vi "250224_Nikon_Control.vi"() -> ()   [LabVIEW 2014]
doc: "This simple VI control few elements of a Nikon Ti2 microscope.\nAny kind of supplementary element can be controlled with a new event type (flurorescence cube turret for example)"
panel:
  in  "Cluster commandes":T1={"Dia lamp"=TRUE, "Dia lamp intensity"=1689.1304347826087, "Objective"=2, "Light path"=2, "Z pos (µm)"=335593, "Filter wheel 2"=2, "Filter wheel 1"=2, "Shutter 2"=TRUE, "Shutter 1"=TRUE} {"Filter wheel 1" items=["1"=1, "2"=2, "3"=3, "4"=4, "5"=5, "6"=6]; "Filter wheel 2" items=["1"=1, "2"=2, "3"=3, "4"=4, "5"=5, "6"=6]; "Z pos (µm)" min=0 max=990000 step=100 scale=0.0..990000.0; "Light path" items=["1- Eyepiece"=1, "2- Right"=2, "3- Left + Eyepiece"=3, "4- Left"=4]; "Objective" items=["1- PLAN APO 100X 1,45 Oil"=1, "2- Empty"=2, "3- Empty"=3, "4- Empty"=4, "5- Empty"=5, "6- Empty"=6]; "Dia lamp intensity" scale=0.0..2100.0}
  out "Cluster µscope":T2
  in  "stop":bool
  in  "NikonTi2AxLib.INikonTi2AxMicroscope":refnum<k7>
  out "error out":errorcluster={"status"=TRUE, "code"=-9, "source"="Exception occured in Nikon.Ti2.Microscope.1: Failed in 231026_NikonTi2_Indicators_v2.vi"} caption="sortie d'erreur"
  in  "error in":errorcluster caption="entrée d'erreur"
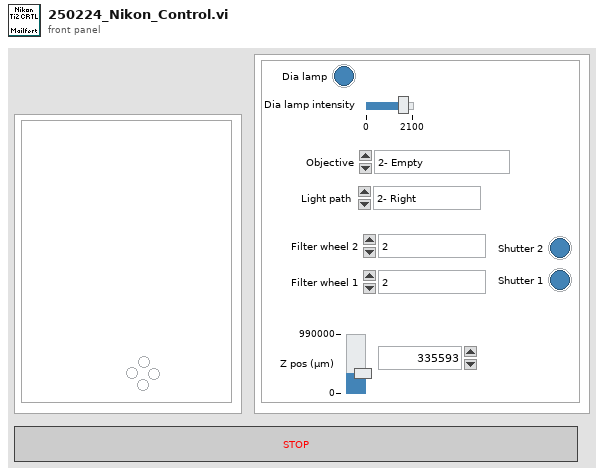
[diagram p1: front panel]
types:
  T1 = cluster{"Dia lamp":bool, "Dia lamp intensity":dbl, "Objective":i32, "Light path":u32, "Z pos (µm)":i32, "Filter wheel 2":u32, "Filter wheel 1":u32, "Shutter 2":bool, "Shutter 1":bool}
  T2 = cluster{"Eyepiece":bool, "Right":bool, "Left + Eyepiece":bool, "Left":bool}
  T3 = cluster{"iNOSEPIECE":i32, "iLIGHTPATH":i32, "iDIA_LAMP_Switch":i32, "iDIA_LAMP_Pos":i32, "iZPOSITION":i32, "iPFS_SWITCH":i32, "iPFS_STATUS":i32, "iPFS_OFFSET":i32, "iTURRET2POS":i32, "Turret2SHUTTER":i32, "iTURRET1POS":i32, "Turret1SHUTTER":i32}
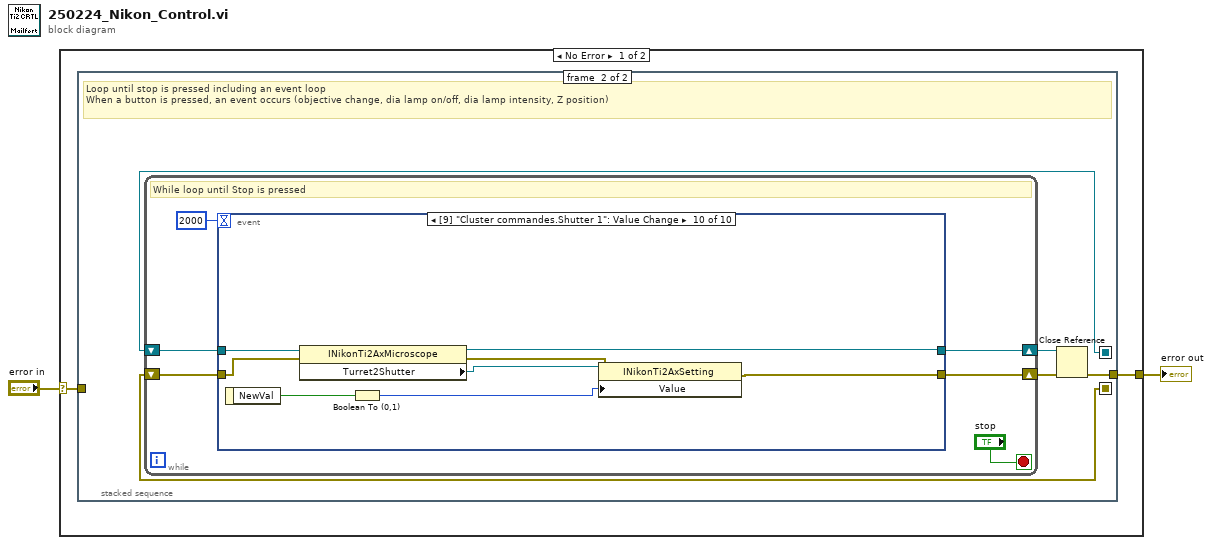
[diagram p0: block diagram]
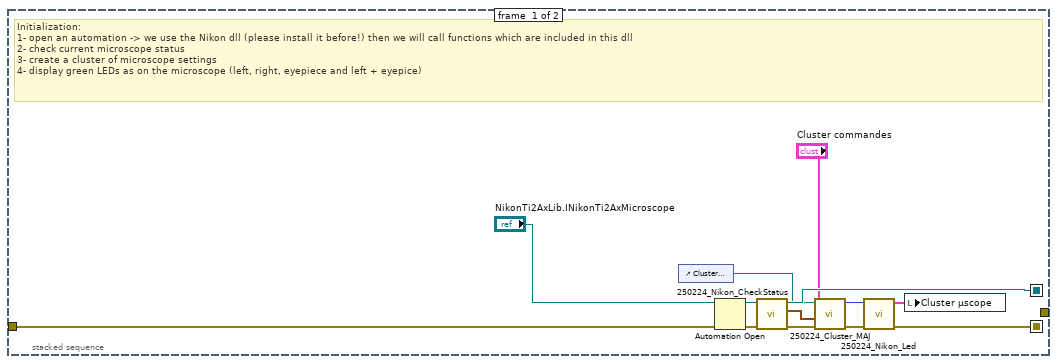
[diagram p2: hidden frame]
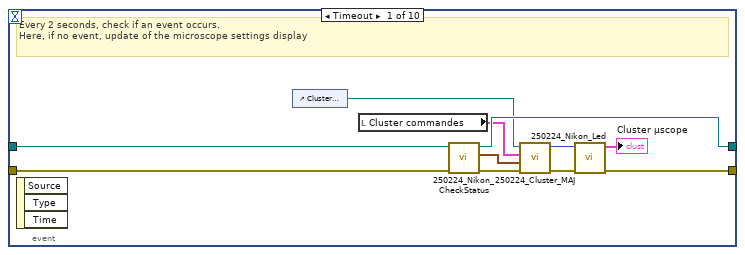
[diagram p3: hidden frame]
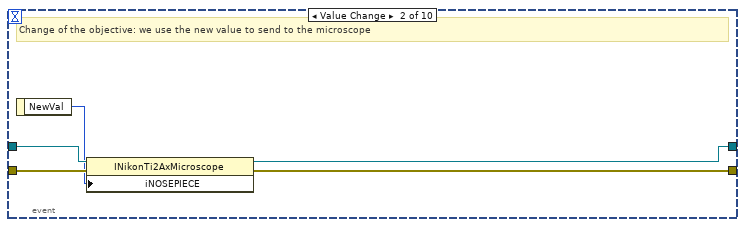
[diagram p4: hidden frame]
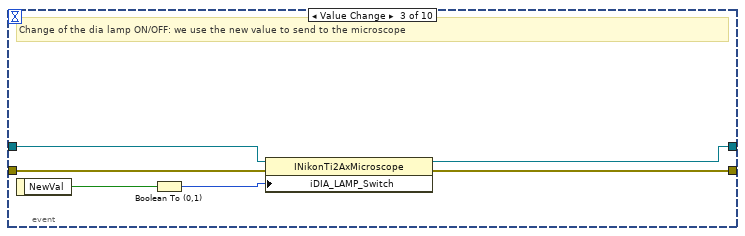
[diagram p5: hidden frame]
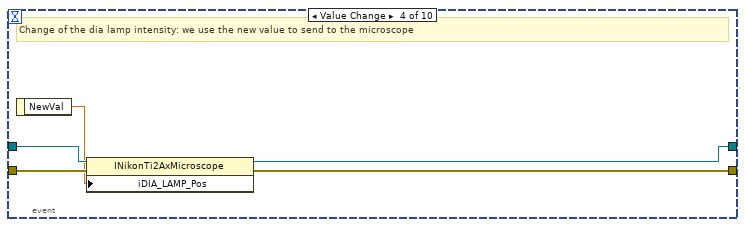
[diagram p6: hidden frame]
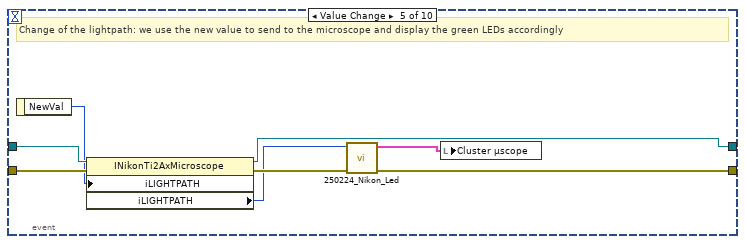
[diagram p7: hidden frame]
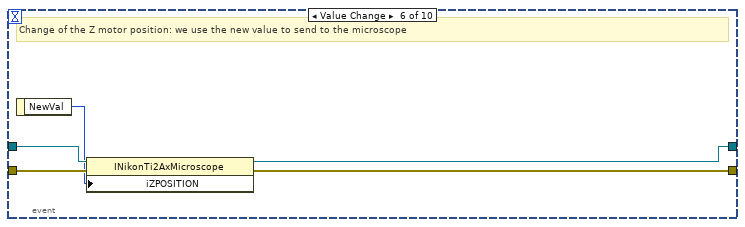
[diagram p8: hidden frame]
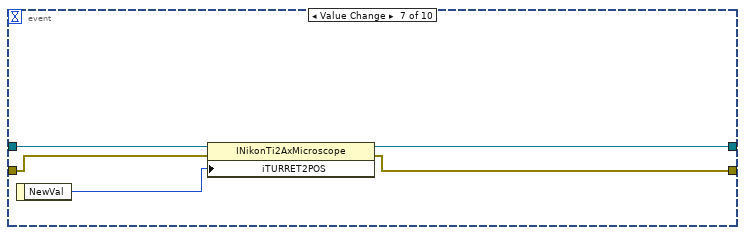
[diagram p9: hidden frame]
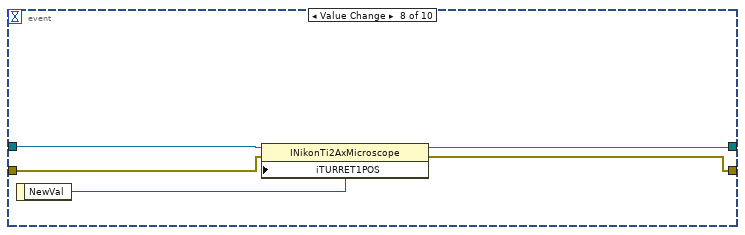
[diagram p10: hidden frame]
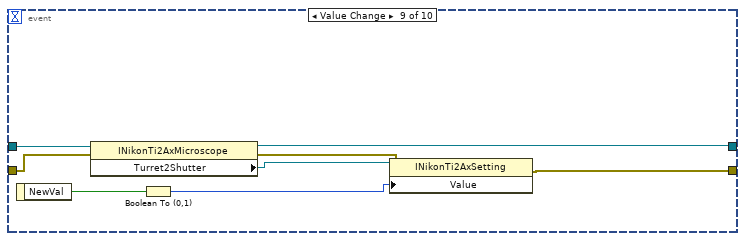
[diagram p11: hidden frame]
diagram:
  n1 = case shown="No Error" "error in" {
    selector: "error in" -> [w4 w95]
    tunnel: [w3 w95] -> w1
    frame No Error {
      n2 = stacked-sequence {
        seq-local: [w13 _] -> [_ w22]
        seq-local: [w7 _] -> [_ w18]
        tunnel: w4 -> [w14 _]
        tunnel: [_ w19] -> w3
        frame #0 {
          # "Initialization:\n1- open an automation -> we use the Nikon dll (please install it before!) then we will call functions which are included in this dll\n2- check current microscope status\n3- create a cluster of microscope settings\n4- display green LEDs as on the microscope (left, right, eyepiece and left + eyepice)"
          n3 = control-ref of="Cluster commandes"() -> (w6:refnum<vi>)
          n4 = Automation Open(error in (no error)=w14, Automation Refnum="NikonTi2AxLib.INikonTi2AxMicroscope") -> (Automation Refnum=w16:refnum<k7>, error out=w15:errorcluster)  [unwired: 2 in]
          n5 = call "250224_Nikon_CheckStatus.vi"("error in"=w15, "NikonTi2AxLib.INikonTi2AxMicroscope"=w16) -> ("error out"=w9:errorcluster, "Nikon status cluster"=w12:T3, "reference out"=w13:refnum<k7>)  [unwired: 7 in]
          n6 = call "250224_Cluster_MAJ.vi"("error in (no error)"=w9, "Nikon status cluster"=w12, 10:"Cluster commandes"="Cluster commandes", 11:"Cluster commandes"=w6) -> ("error out"=w8:errorcluster, "iLIGHTPATH"=w10:i32)  [unwired: 6 in]
          n7 = call "250224_Nikon_Led.vi"("error in"=w8, "Light path"=w10) -> ("error out"=w7:errorcluster, "Cluster µscope"=w11:T2)  [unwired: 8 in]
          n8 = local write "Cluster µscope"(w11) -> ()
        }
        frame #1 {
          # "Loop until stop is pressed including an event loop\nWhen a button is pressed, an event occurs (objective change, dia lamp on/off, dia lamp intensity, Z position)"
          n9 = while {
            shift-right: [w23] -> w20
            shift-left: w18 -> [w28]
            shift-right: [w24] -> w21
            shift-left: w22 -> [w25]
            stop <- "stop" stop-if-true
            # "While loop until Stop is pressed"
            n10 = event shown="[9] \"Cluster commandes.Shutter 1\": Value Change" {
              selector: _ -> [_ _ _ _ _ _ _ _ _ _]
              dyn-events: _ -> [_ _ _ _ _ _ _ _ _ _]
              timeout: 2000 -> [_ _ _ _ _ _ _ _ _ _]
              tunnel: [w36 w41 w47 w52 w60 w67 w70 w74 w81 w89] -> w23
              tunnel: w28 -> [w39 w43 w49 w54 w61 w65 w71 w77 w86 w94]
              tunnel: w25 -> [w38 w44 w50 w55 w62 w66 w73 w78 w85 w93]
              tunnel: [w37 w42 w48 w53 w63 w68 w69 w75 w82 w90] -> w24
              event Timeout {
                # "Every 2 seconds, check if an event occurs.\nHere, if no event, update of the microscope settings display"
                n11 = event-data() -> ()  [unwired: 1 in, 3 out]
                n12 = control-ref of="Cluster commandes"() -> (w29:refnum<vi>)
                n13 = local read "Cluster commandes"() -> (w30:T1)
                n14 = call "250224_Nikon_CheckStatus.vi"("error in"=w39, "NikonTi2AxLib.INikonTi2AxMicroscope"=w38) -> ("error out"=w33:errorcluster, "Nikon status cluster"=w34:T3, "reference out"=w37:refnum<k7>)  [unwired: 7 in]
                n15 = call "250224_Cluster_MAJ.vi"("error in (no error)"=w33, "Nikon status cluster"=w34, 10:"Cluster commandes"=w30, 11:"Cluster commandes"=w29) -> ("error out"=w32:errorcluster, "iLIGHTPATH"=w31:i32)  [unwired: 6 in]
                n16 = call "250224_Nikon_Led.vi"("error in"=w32, "Light path"=w31) -> ("error out"=w36:errorcluster, "Cluster µscope"=→"Cluster µscope":T2)  [unwired: 8 in]
              }
              event "Cluster commandes.Objective": Value Change {
                # "Change of the objective: we use the new value to send to the microscope"
                n17 = event-data() -> ("NewVal"=w40:i32)  [unwired: 1 in]
                n18 = property class="INikonTi2AxMicroscope"(reference=w44, error in=w43, "iNOSEPIECE"=w40) -> (reference out=w42:refnum<k7>, error out=w41:errorcluster)
              }
              event "Cluster commandes.Dia lamp": Value Change {
                # "Change of the dia lamp ON/OFF: we use the new value to send to the microscope"
                n19 = event-data() -> ("NewVal"=w46:bool)  [unwired: 1 in]
                n20 = Boolean To (0,1)(Boolean=w46) -> (0, 1=w45:i16)
                n21 = property class="INikonTi2AxMicroscope"(reference=w50, error in=w49, "iDIA_LAMP_Switch"=w45) -> (reference out=w48:refnum<k7>, error out=w47:errorcluster)
              }
              event "Cluster commandes.Dia lamp intensity": Value Change {
                # "Change of the dia lamp intensity: we use the new value to send to the microscope"
                n22 = event-data() -> ("NewVal"=w51:dbl)  [unwired: 1 in]
                n23 = property class="INikonTi2AxMicroscope"(reference=w55, error in=w54, "iDIA_LAMP_Pos"=w51) -> (reference out=w53:refnum<k7>, error out=w52:errorcluster)
              }
              event "Cluster commandes.Light path": Value Change {
                # "Change of the lightpath: we use the new value to send to the microscope and display the green LEDs accordingly"
                n24 = event-data() -> ("NewVal"=w57:u32)  [unwired: 1 in]
                n25 = property class="INikonTi2AxMicroscope"(reference=w62, error in=w61, "iLIGHTPATH"=w57) -> (reference out=w63:refnum<k7>, error out=w59:errorcluster, "iLIGHTPATH"=w58:i32)
                n26 = call "250224_Nikon_Led.vi"("error in"=w59, "Light path"=w58) -> ("error out"=w60:errorcluster, "Cluster µscope"=w56:T2)  [unwired: 8 in]
                n27 = local write "Cluster µscope"(w56) -> ()
              }
              event "Cluster commandes.Z pos (µm)": Value Change {
                # "Change of the Z motor position: we use the new value to send to the microscope"
                n28 = event-data() -> ("NewVal"=w64:i32)  [unwired: 1 in]
                n29 = property class="INikonTi2AxMicroscope"(reference=w66, error in=w65, "iZPOSITION"=w64) -> (reference out=w68:refnum<k7>, error out=w67:errorcluster)
              }
              event "Cluster commandes.Filter wheel 2": Value Change {
                n30 = event-data() -> ("NewVal"=w72:u32)  [unwired: 1 in]
                n31 = property class="INikonTi2AxMicroscope"(reference=w73, error in=w71, "iTURRET2POS"=w72) -> (reference out=w69:refnum<k7>, error out=w70:errorcluster)
              }
              event "Cluster commandes.Filter wheel 1": Value Change {
                n32 = event-data() -> ("NewVal"=w76:u32)  [unwired: 1 in]
                n33 = property class="INikonTi2AxMicroscope"(reference=w78, error in=w77, "iTURRET1POS"=w76) -> (reference out=w75:refnum<k7>, error out=w74:errorcluster)
              }
              event "Cluster commandes.Shutter 2": Value Change {
                n34 = event-data() -> ("NewVal"=w80:bool)  [unwired: 1 in]
                n35 = property class="INikonTi2AxMicroscope"(reference=w85, error in=w86) -> (reference out=w82:refnum<k7>, error out=w83:errorcluster, "Turret2Shutter"=w84:refnum<k7>)
                n36 = Boolean To (0,1)(Boolean=w80) -> (0, 1=w79:i16)
                n37 = property class="INikonTi2AxSetting"(reference=w84, error in=w83, "Value"=w79) -> (error out=w81:errorcluster)  [unwired: 1 out]
              }
              event "Cluster commandes.Shutter 1": Value Change {
                n38 = event-data() -> ("NewVal"=w88:bool)  [unwired: 1 in]
                n39 = property class="INikonTi2AxMicroscope"(reference=w93, error in=w94) -> (reference out=w90:refnum<k7>, error out=w91:errorcluster, "Turret2Shutter"=w92:refnum<k7>)
                n40 = Boolean To (0,1)(Boolean=w88) -> (0, 1=w87:i16)
                n41 = property class="INikonTi2AxSetting"(reference=w92, error in=w91, "Value"=w87) -> (error out=w89:errorcluster)  [unwired: 1 out]
              }
            }
          }
          n42 = Close Reference(reference=w21, error in (no error)=w20) -> (error out=w19:errorcluster)
        }
      }
    }
    frame Error {
    }
  }
  "error out" <- w1
